vi "CurrentItem.vi"(0 "object in":refnum<class "DFSTreeIterator.lvclass">, 5 "Error In":errorcluster) -> (14 "object out":refnum<class "DFSTreeIterator.lvclass">, 16 "Current Item":refnum<class "Node.lvclass">, 19 "Error Out":errorcluster)   [LabVIEW 2024, in "DFSTreeIterator.lvclass"]
uses:
  DFSTreeIterator.lvclass
  Node_class/Node.lvclass
  DFSTreeIterator.lvclass/DFSTreeIterator.ctl
  Support/Stack_class/Stack.lvclass
panel:
  # "Connector Pane"
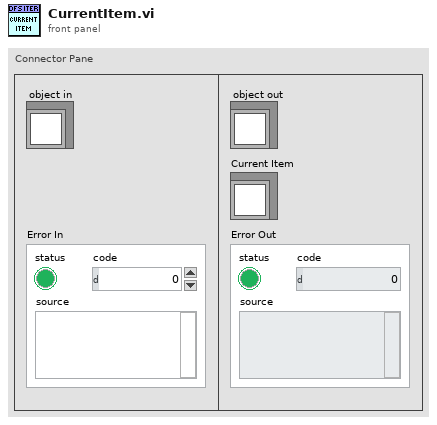
[diagram p1: front panel]
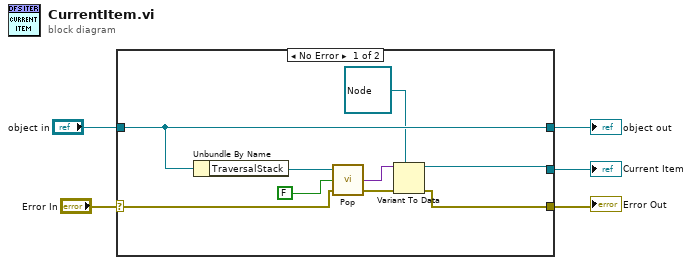
[diagram p0: block diagram]
diagram:
  n1 = case shown="No Error" "Error In" {
    selector: "Error In" -> [w14 w16]
    tunnel: [w9 w16] -> w4
    tunnel: [w13 w15] -> w2
    tunnel: "object in" -> [w13 w15]
    tunnel: [w8 _] -> w1
    frame No Error {
      n2 = Unbundle By Name(w13) -> ("TraversalStack"=w11:refnum<class "Stack.lvclass">)
      n3 = call-dynamic "Pop.vi"("Error In"=w14, "Delete?"=FALSE, "object in"=w11) -> ("Error Out"=w12:errorcluster, "Data"=w7:variant)  [unwired: 1 out]
      n4 = Variant To Data(error in=w12, type=refnum<class "Node.lvclass"> refnum ("Node"), Variant=w7) -> (data=w8:refnum<class "Node.lvclass">, error out=w9:errorcluster)
    }
    frame Error {
    }
  }
  "Error Out" <- w4
  "object out" <- w2
  "Current Item" <- w1
